vi "EE Calculation.vi"() -> ()   [LabVIEW 2009]
panel:
  out "BMR":dbl
  out "EE":dbl
  in  "Compcode":i32
  in  "MET":dbl
  in  "Sex (1=Male, 0=Female)":dbl
  in  "Age":dbl
  in  "Height (cm)":dbl
  in  "Weight (Kg)":dbl
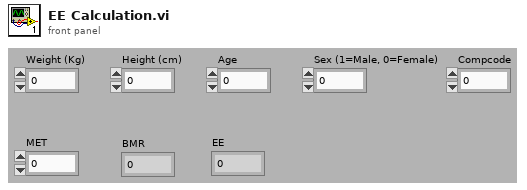
[diagram p1: front panel]
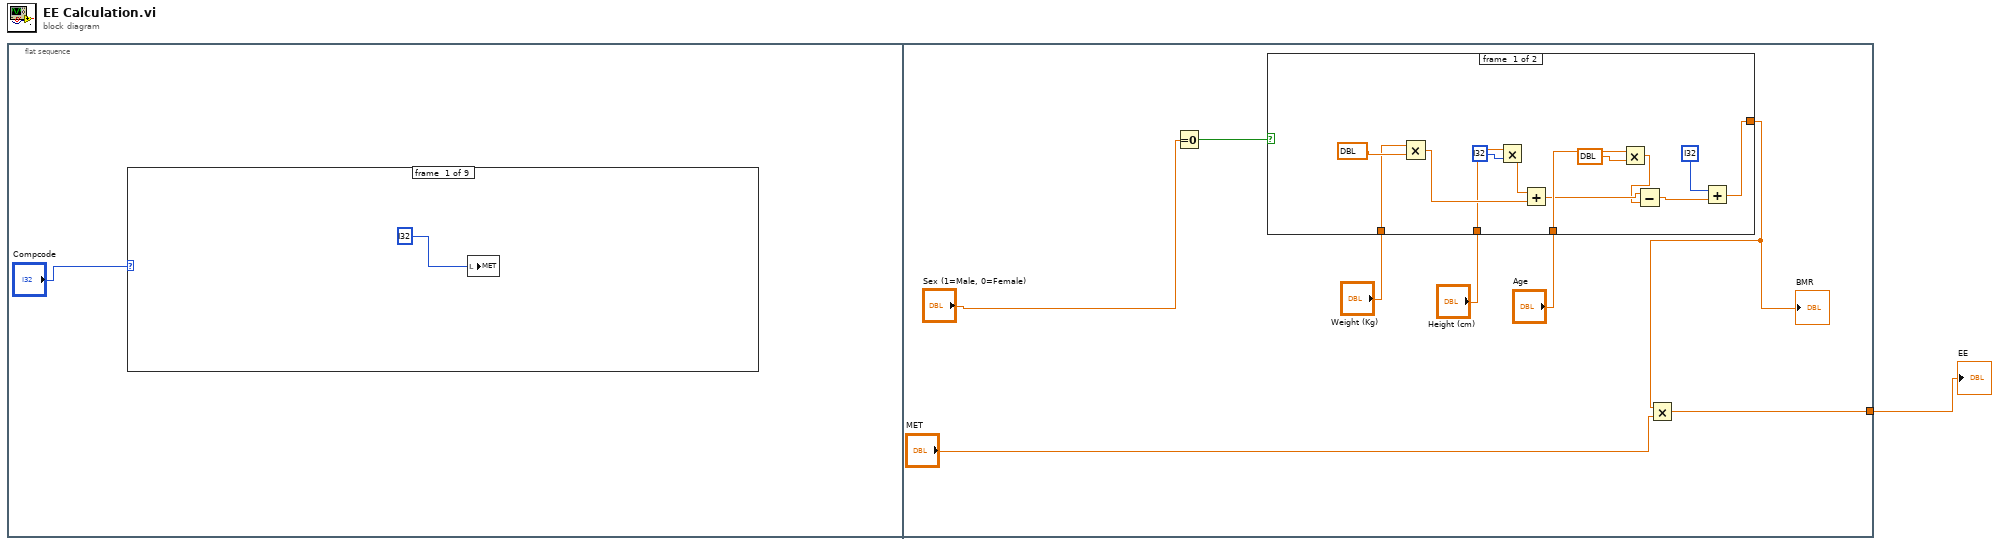
[diagram p0: block diagram]
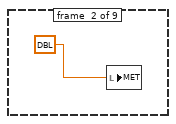
[diagram p2: hidden frame]
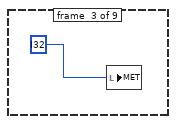
[diagram p3: hidden frame]
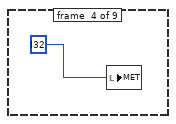
[diagram p4: hidden frame]
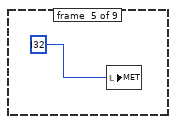
[diagram p5: hidden frame]
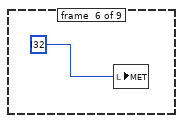
[diagram p6: hidden frame]
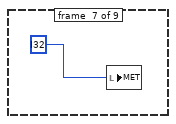
[diagram p7: hidden frame]
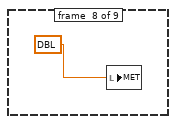
[diagram p8: hidden frame]
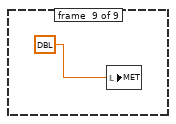
[diagram p9: hidden frame]
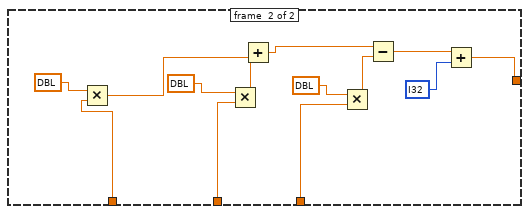
[diagram p10: hidden frame]
diagram:
  n1 = flat-sequence {
    tunnel: [w13] -> w1
    frame #0 {
      n2 = case shown="7040" "Compcode" {
        frame #0 {
          n3 = local write "MET"(i32 ?) -> ()
        }
        frame #1 {
          n4 = local write "MET"(dbl ?) -> ()
        }
        frame #2 {
          n5 = local write "MET"(i32 ?) -> ()
        }
        frame #3 {
          n6 = local write "MET"(i32 ?) -> ()
        }
        frame #4 {
          n7 = local write "MET"(i32 ?) -> ()
        }
        frame #5 {
          n8 = local write "MET"(i32 ?) -> ()
        }
        frame #6 {
          n9 = local write "MET"(i32 ?) -> ()
        }
        frame #7 {
          n10 = local write "MET"(dbl ?) -> ()
        }
        frame #8 {
          n11 = local write "MET"(dbl ?) -> ()
        }
      }
    }
    frame #1 {
      n12 = Equal To 0?(x="Sex (1=Male, 0=Female)") -> (x = 0?=w15:bool)
      n13 = case shown="True" w15 {
        tunnel: "Weight (Kg)" -> [w25 w45]
        tunnel: "Height (cm)" -> [w24 w43]
        tunnel: "Age" -> [w23 w40]
        tunnel: [w22 w33] -> w12
        frame #0 {
          n14 = Multiply(x=w25, y=dbl ?) -> (x*y=w29:dbl)
          n15 = Multiply(x=w24, y=i32 ?) -> (x*y=w28:dbl)
          n16 = Add(x=w28, y=w29) -> (x+y=w21:dbl)
          n17 = Multiply(x=w23, y=dbl ?) -> (x*y=w20:dbl)
          n18 = Subtract(x=w21, y=w20) -> (x-y=w27:dbl)
          n19 = Add(x=i32 ?, y=w27) -> (x+y=w22:dbl)
        }
        frame #1 {
          n20 = Multiply(x=dbl ?, y=w45) -> (x*y=w39:dbl)
          n21 = Multiply(x=dbl ?, y=w43) -> (x*y=w38:dbl)
          n22 = Add(x=w38, y=w39) -> (x+y=w37:dbl)
          n23 = Multiply(x=dbl ?, y=w40) -> (x*y=w36:dbl)
          n24 = Subtract(x=w37, y=w36) -> (x-y=w34:dbl)
          n25 = Add(x=w34, y=i32 ?) -> (x+y=w33:dbl)
        }
      }
      "BMR" <- w12
      n26 = Multiply(x=w12, y="MET") -> (x*y=w13:dbl)
    }
  }
  "EE" <- w1
